vi "SIP_day00204.vi"(4 "Enum":enum16{"Morlet Wavelet", "damp sine"}(ring), 5 "noise":bool, 6 "Shift":dbl(slide) scale=0.0..1000.0, 7 "B factor":dbl(slide) scale=0.0..1000.0, 8 "N 2":i32(slide) scale=0.0..1000.0, 9 "Amplitude A 2":dbl(slide) scale=0.0..10.0, 10 "NP 2":dbl(slide) scale=0.0..10.0, 11 "SD":dbl(slide) scale=0.0..10.0) -> (3 "Waveform Graph 2":dbl[](graph))   [LabVIEW 2025]
uses:
  <vilib>/Analysis/NI_AALBase.lvlib
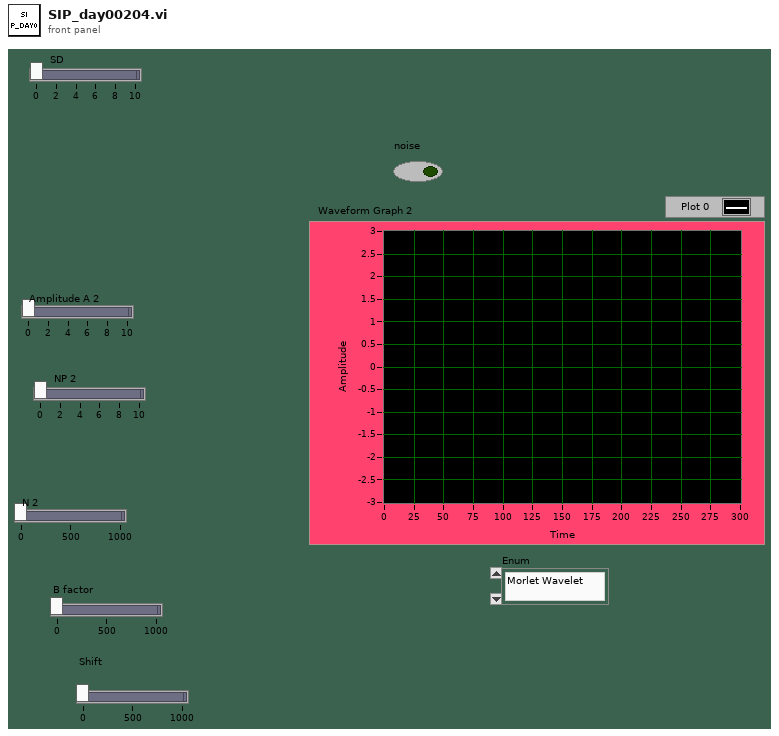
[diagram p1: front panel]
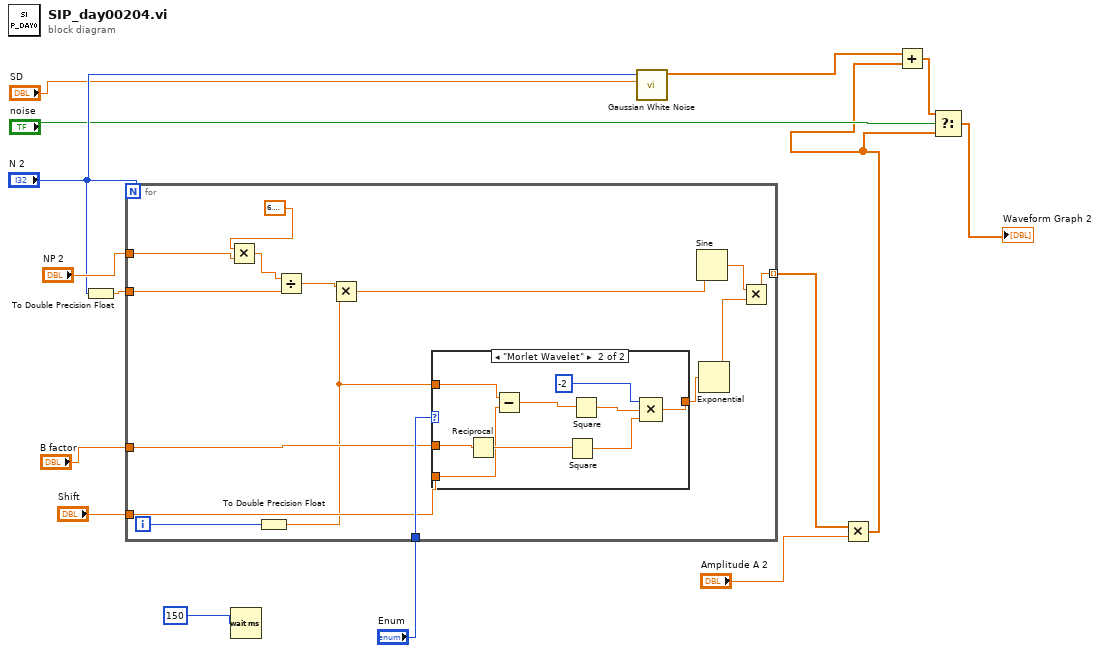
[diagram p0: block diagram]
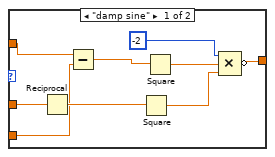
[diagram p2: hidden frame]
diagram:
  n1 = To Double Precision Float(number="N 2") -> (double precision float=w14:dbl)
  n2 = for {
    N: "N 2" -> [_]
    tunnel: "NP 2" -> [w30]
    tunnel: w14 -> [w28]
    tunnel: [w18] -> w12 mode=indexing
    tunnel: "Enum" -> [w23]
    tunnel: "B factor" -> [w22]
    tunnel: "Shift" -> [w17]
    i -> [w26]
    n3 = Multiply(x=6.283185307179586, y=w30) -> (x*y=w29:dbl)
    n4 = To Double Precision Float(number=w26) -> (double precision float=w16:dbl)
    n5 = Divide(x=w29, y=w28) -> (x/y=w27:dbl)
    n6 = Multiply(x=w27, y=w16) -> (x*y=w25:dbl)
    n7 = case shown="\"Morlet Wavelet\"" w23 {
      tunnel: w16 -> [w35 w42]
      tunnel: w22 -> [w39 w41]
      tunnel: [w31 w43] -> w21
      tunnel: w17 -> [w34 w40]
      frame "damp sine" {
        n8 = Reciprocal(x=w39) -> (1/x=w38:dbl)
        n9 = Subtract(x=w35, y=w34) -> (x-y=w33:dbl)
        n10 = Square(x=w38) -> (x^2=w37:dbl)
        n11 = Square(x=w33) -> (x^2=w32:dbl)
        n12 = Compound Arithmetic op=MULTIPLY(-2, w32, w37) -> (invert w31:dbl)
      }
      frame "Morlet Wavelet" {
        n13 = Reciprocal(x=w41) -> (1/x=w48:dbl)
        n14 = Subtract(x=w42, y=w40) -> (x-y=w45:dbl)
        n15 = Square(x=w48) -> (x^2=w47:dbl)
        n16 = Square(x=w45) -> (x^2=w44:dbl)
        n17 = Compound Arithmetic op=MULTIPLY(-2, w44, w47) -> (w43:dbl)
      }
    }
    n18 = Sine(x=w25) -> (sin(x)=w20:dbl)
    n19 = Exponential(1:w21) -> (0:w19:dbl)
    n20 = Multiply(x=w20, y=w19) -> (x*y=w18:dbl)
  }
  n21 = Wait (ms)(milliseconds to wait=u32 150 ("millisecond timer value")) -> ()  [unwired: 1 out]
  n22 = call <vilib>:"Gaussian White Noise.vi"("standard deviation"="SD", "samples"="N 2") -> ("Gaussian noise pattern"=w6:dbl[])  [unwired: 8 in, 1 out]
  n23 = Multiply(x=w12, y="Amplitude A 2") -> (x*y=w4:dbl[])
  n24 = Add(x=w6, y=w4) -> (x+y=w2:dbl[])
  n25 = Select(t=w2, s="noise", f=w4) -> (s? t:f=→"Waveform Graph 2":dbl[])
